vi "PlaySound.vi"(8 "error in (no error)":errorcluster, 9 "Overwrite":bool, 10 "Name":string) -> (0 "error out":errorcluster)   [LabVIEW 2019, in "RT_Game.lvlib" / "Engine.lvclass"]
uses:
  Engine.lvclass
  MessageCluster.ctl
  PlaySoundData.ctl
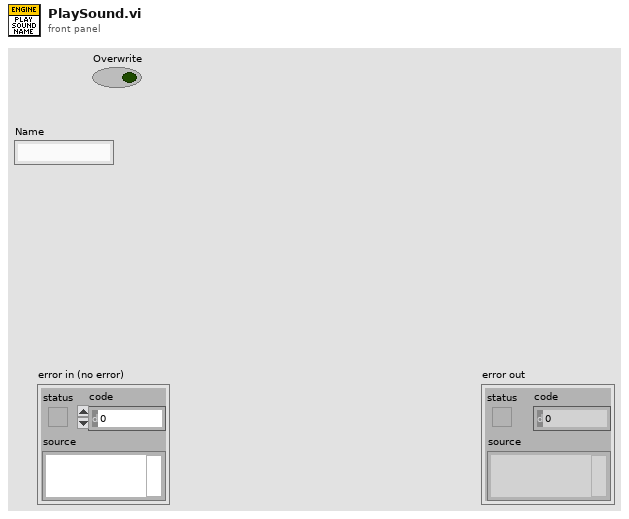
[diagram p1: front panel]
types:
  T1 = typedef "RT_Game.lvlib/Engine.lvclass/PlaySoundData.ctl" = cluster{"Name":string, "Overwrite":bool}
  T2 = typedef "RT_Game.lvlib/Engine.lvclass/MessageCluster.ctl" = cluster{"Message":string, "Data":variant}
  T3 = typedef "RT_Game.lvlib/Engine.lvclass/Queues.ctl" = cluster{"MusicQueue":refnum<queue>, "TilesQueue":refnum<queue>, "SoundsQueue":refnum<queue>}
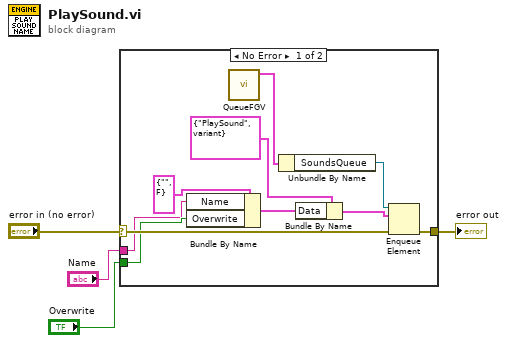
[diagram p0: block diagram]
diagram:
  n1 = case shown="No Error" "error in (no error)" {
    selector: "error in (no error)" -> [w14 w15]
    tunnel: [w13 w15] -> w3
    tunnel: "Overwrite" -> [w7 _]
    tunnel: "Name" -> [w6 _]
    frame No Error {
      n2 = Bundle By Name(cluster=T1 {"Name"="", "Overwrite"=FALSE} ("PlaySoundData"), "Name"=w6, "Overwrite"=w7) -> (w8:T1)
      n3 = call "QueueFGV.vi"() -> ("Queues out"=w5:T3)  [unwired: 10 in, 1 out]
      n4 = Unbundle By Name(w5) -> ("SoundsQueue"=w12:refnum<queue>)
      n5 = Bundle By Name(cluster=T2 {"Message"="PlaySound", "Data"=variant} ("element"), "Data"=w8) -> (w10:T2)
      n6 = Enqueue Element(queue=w12, element=w10, error in (no error)=w14) -> (error out=w13:errorcluster)  [unwired: 1 in, 2 out]
    }
    frame Error {
    }
  }
  "error out" <- w3
